vi "GDFdisplayNextDataset.vi"(0 "data value reference in":refnum<data-value>, 5 "Start":dbl format="%0.2f", 7 "Duration":dbl format="%0.2f", 9 "Waveform Graph Refnum in":refnum<vi>, 11 "error in (no error)":errorcluster, 12 "start/duration format":u16(ring)=1 items=["Samples", "Relative Time"]) -> (4 "data value reference out":refnum<data-value>, 15 "error out":errorcluster)   [LabVIEW 2016, in "GDF File Reader.lvlib"]
uses:
  <vilib>/Waveform/WDTOps.llb/WDT Get Waveform Subset DBL.vi
  GDF File Reader.lvlib
panel:
  # "This VI is a part of BCI Design library, http://www.ru-bci.org \nCopyright © 2020, Sotnikov Peter, All rights reserved. License: GNU GPLv3"
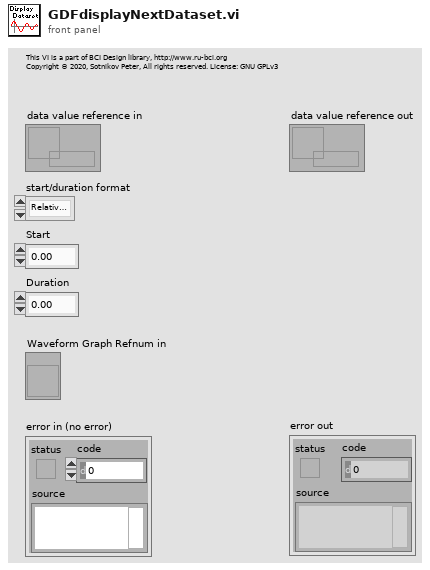
[diagram p1: front panel]
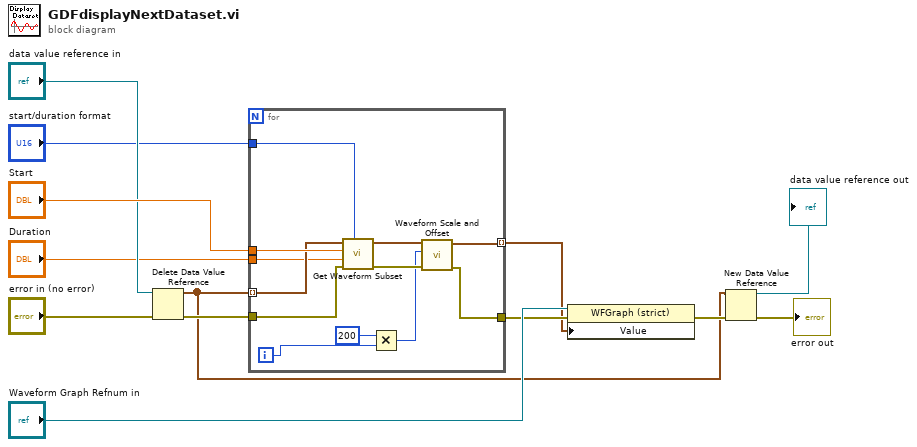
[diagram p0: block diagram]
diagram:
  n1 = Delete Data Value Reference(data value reference="data value reference in", error in="error in (no error)") -> (data value=w2:waveform(dbl)[], error out=w7:errorcluster)
  n2 = for {
    tunnel: [w15] -> w10 mode=indexing
    tunnel: "Start" -> [w25]
    tunnel: w7 -> [w24]
    tunnel: [w14] -> w11
    tunnel: w2 -> [w23] mode=indexing
    tunnel: "start/duration format" -> [w22]
    tunnel: "Duration" -> [w21]
    i -> [w18]
    n3 = call-poly <vilib>:"Get Waveform Subset.vi"("start/duration format"=w22, "error in (no error)"=w24, "duration"=w21, "start samples/time"=w25, "waveform in"=w23) -> ("error out"=w20:errorcluster, "waveform out"=w19:waveform(dbl))  [unwired: 1 in, 2 out]
    n4 = Multiply(x=200, y=w18) -> (x*y=w16:i32)
    n5 = call <vilib>:"Waveform Scale and Offset.vi"("error in (no error)"=w20, "offset"=w16, "waveform in"=w19) -> ("error out"=w14:errorcluster, "waveform out"=w15:waveform(dbl))  [unwired: 7 in]
  }
  n6 = property class="WFGraph (strict)"(reference="Waveform Graph Refnum in", error in=w11, "Value"=w10) -> (error out=w4:errorcluster)  [unwired: 1 out]
  n7 = New Data Value Reference(data value=w2, error in=w4) -> (data value reference=→"data value reference out":refnum<data-value>, error out=→"error out":errorcluster)
